vi "Plot Maximize Button.vi"(7 "VI ref":refnum<vi>, 8 "error in (no error)":errorcluster, 9 "max button reference":refnum<vi>, 10 "NewVal":bool, 11 "BluePlotHandle in":refnum<class "RocketPlotHandle.lvclass">) -> (0 "error out":errorcluster, 3 "BluePlotHandle out":refnum<class "RocketPlotHandle.lvclass">)   [LabVIEW 2021, in "RocketPlotHandle.lvclass"]
uses:
  RocketPlotHandle.lvclass
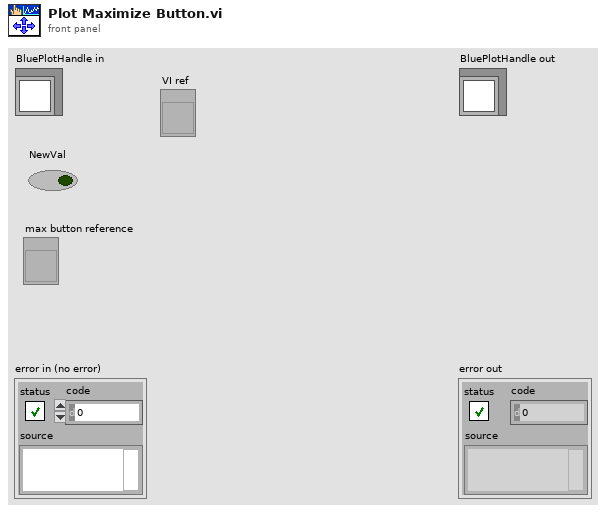
[diagram p1: front panel]
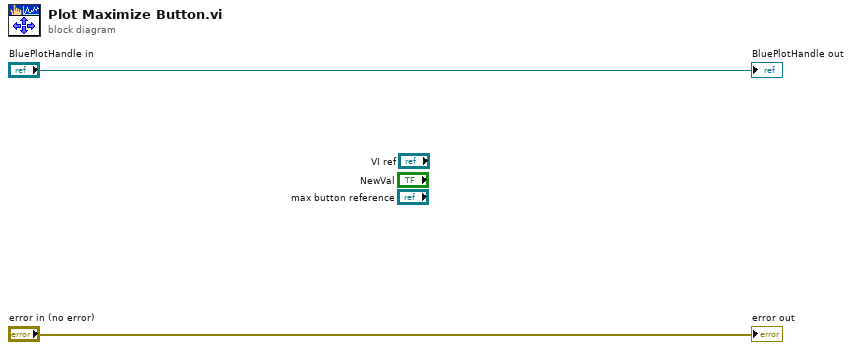
[diagram p0: block diagram]
diagram:
  "error out" <- "error in (no error)"
  "BluePlotHandle out" <- "BluePlotHandle in"
